vi "ADCP_UI_Continuous_Receiver_Data_Packet_Updater.vi"(8 "error in (no error)":errorcluster, 11 "ADCU_GUI References":T1) -> ()   [LabVIEW 2017]
uses:
  Controls/ADCP_UI/ADCP_UI_Parameters.ctl
  Controls/ADCP_UI/ADCP_UI_Queues.ctl
  Controls/ADCP_UI/ADCP_UI_Continuous_Receiver_States.ctl
  Controls/ADCP_UI/ADCP_Queue_Receive_Log_Queue_Element.ctl
  Controls/Packet/Packet.ctl
  Controls/Packet/Packet_Direction.ctl
  Controls/Packet/Packet_Type.ctl
  Controls/Packet/Packet_Priority.ctl
  Controls/Data Packets/Data_Packet.ctl
  Controls/Data Packets/Parameter.ctl
  Controls/Data Packets/Parameter_Data_Type.ctl
  Controls/Data Packets/Data_Packet_Transmit_Mode.ctl
  Controls/Data Packets/Data_Packet_FGV_Commands.ctl
  ADCP_UI_Receive_List_Data_Packets.vi
panel:
  out "Packet.Frame ID":u8
  out "Packet.Node ID":u8
  out "Process Data":bool
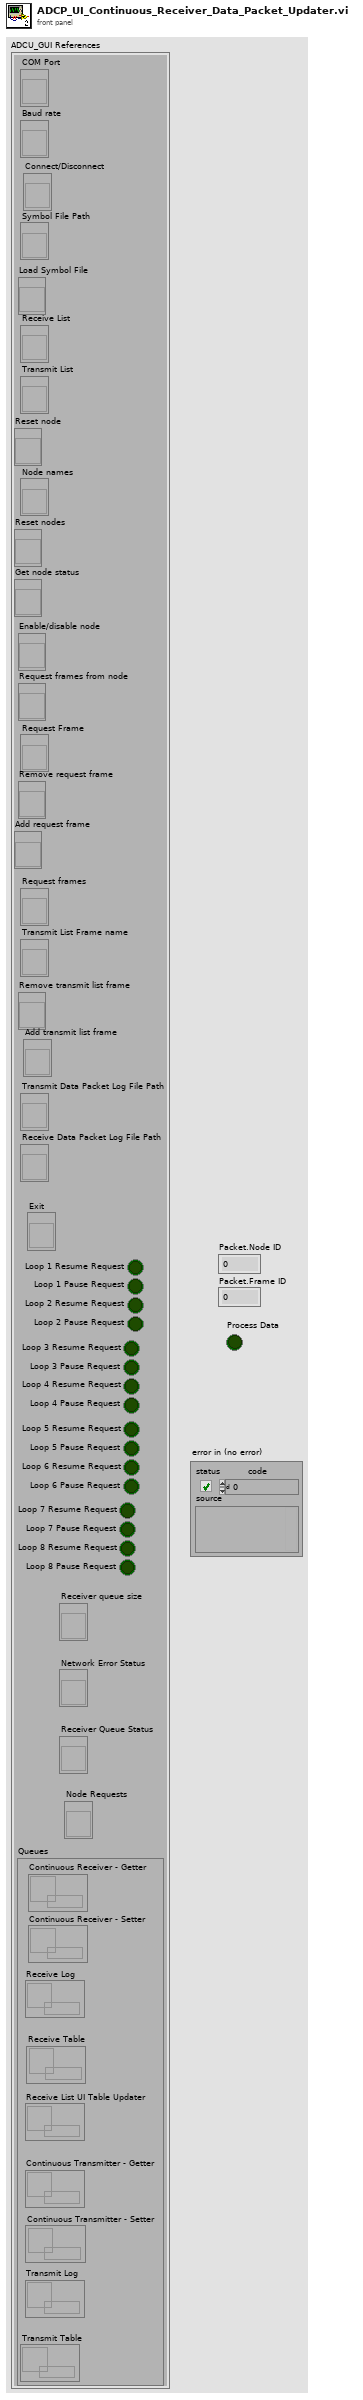
[diagram p1: front panel]
types:
  T1 = typedef "ADCP_UI_Parameters.ctl" = cluster{"COM Port":refnum<vi>, "Baud rate":refnum<vi>, "Symbol File Path":refnum<vi>, "Receive List":refnum<vi>, "Transmit List":refnum<vi>, "Node names":refnum<vi>, "Request Frame":refnum<vi>, "Request frames":refnum<vi>, "Transmit List Frame name":refnum<vi>, "Transmit Data Packet Log File Path":refnum<vi>, "Receive Data Packet Log File Path":refnum<vi>, "Loop 1 Resume Request":bool, "Loop 1 Pause Request":bool, "Loop 2 Resume Request":bool, "Loop 2 Pause Request":bool, "Loop 3 Resume Request":bool, "Loop 3 Pause Request":bool, "Loop 4 Resume Request":bool, "Loop 4 Pause Request":bool, "Loop 5 Resume Request":bool, "Loop 5 Pause Request":bool, "Loop 6 Resume Request":bool, "Loop 6 Pause Request":bool, "Loop 7 Resume Request":bool, "Loop 7 Pause Request":bool, "Loop 8 Resume Request":bool, "Loop 8 Pause Request":bool, "Exit":refnum<vi>, "Connect/Disconnect":refnum<vi>, "Load Symbol File":refnum<vi>, "Reset node":refnum<vi>, "Reset nodes":refnum<vi>, "Get node status":refnum<vi>, "Enable/disable node":refnum<vi>, "Request frames from node":refnum<vi>, "Remove request frame":refnum<vi>, "Add request frame":refnum<vi>, "Remove transmit list frame":refnum<vi>, "Add transmit list frame":refnum<vi>, "Receiver queue size":refnum<vi>, "Network Error Status":refnum<vi>, "Receiver Queue Status":refnum<vi>, "Node Requests":refnum<vi>, "Queues":T2}
  T2 = typedef "ADCP_UI_Queues.ctl" = cluster{"Continuous Receiver - Getter":refnum<queue>, "Continuous Receiver - Setter":refnum<queue>, "Receive Log":refnum<queue>, "Receive Table":refnum<queue>, "Receive List UI Table Updater":refnum<queue>, "Continuous Transmitter - Getter":refnum<queue>, "Continuous Transmitter - Setter":refnum<queue>, "Transmit Log":refnum<queue>, "Transmit Table":refnum<queue>}
  T3 = typedef "Data_Packet_FGV_Commands.ctl" = enum16{"Update all parameters from data packets", "Update Packet", "Load", "Read Packet Parameters", "Write Packet Parameters", "Read Packet Parameter", "Write Packet Parameter", "Read Data Packets", "Read Data Packet", "Read Data Packet by Parameter Name", "Get Parameter Node and Frame ID", "Read Data Packet from Node ID and Frame ID"}
  T4 = typedef "ADCP_Queue_Receive_Log_Queue_Element.ctl" = cluster{"Packet":T5, "Receive Time (ms)":u64, "Count":i32, "Receive Time Interval (ms) ":u64}
  T5 = typedef "Packet.ctl" = cluster{"Raw Bytes":u8[], "Checksum":bool, "Direction":T6, "Processed Bytes":u8[], "Node ID":u8, "Packet type":T7, "Frame Data":u32, "Priority":T8, "Frame ID":u8}
  T6 = typedef "Packet_Direction.ctl" = enum16{"Transmit", "Receive", "Bidirectional"}
  T7 = typedef "Packet_Type.ctl" = enum16{"Data", "Connection Management", "Remote Request", "Error/Status"}
  T8 = typedef "Packet_Priority.ctl" = enum16{"LOW", "HIGH"}
  T9 = typedef "Data_Packet.ctl" = cluster{"Packet":T5, "Parameters":T10[], "Last Received Time (ms)":u64, "Receive count":i32, "Transmit count":i32, "Transmit interval (ms)":u32, "Last Transmitted Time (ms)":u64, "Receive interval (ms)":u32, "Transmit_Mode":T12, "Transmit Enable":bool, "Cyclic Transmit interval (ms)":u32}
  T10 = typedef "Parameter.ctl" = cluster{"Parameter name":string, "Node name":string, "Node ID":u8, "Frame name":string, "Frame ID":u8, "Data type":T11, "Start Bit":i32, "Bit Length":i32, "Factor":dbl, "Offset":dbl, "Minimum":dbl, "Maximum":dbl, "Descriptor":string, "Enum values":string[], "Value":string}
  T11 = typedef "Parameter_Data_Type.ctl" = enum16{"BOOL", "UNSIGNED", "SIGNED", "FLOAT32", "ENUM"}
  T12 = typedef "Data_Packet_Transmit_Mode.ctl" = enum16{"Disabled", "Single", "Cyclic"}
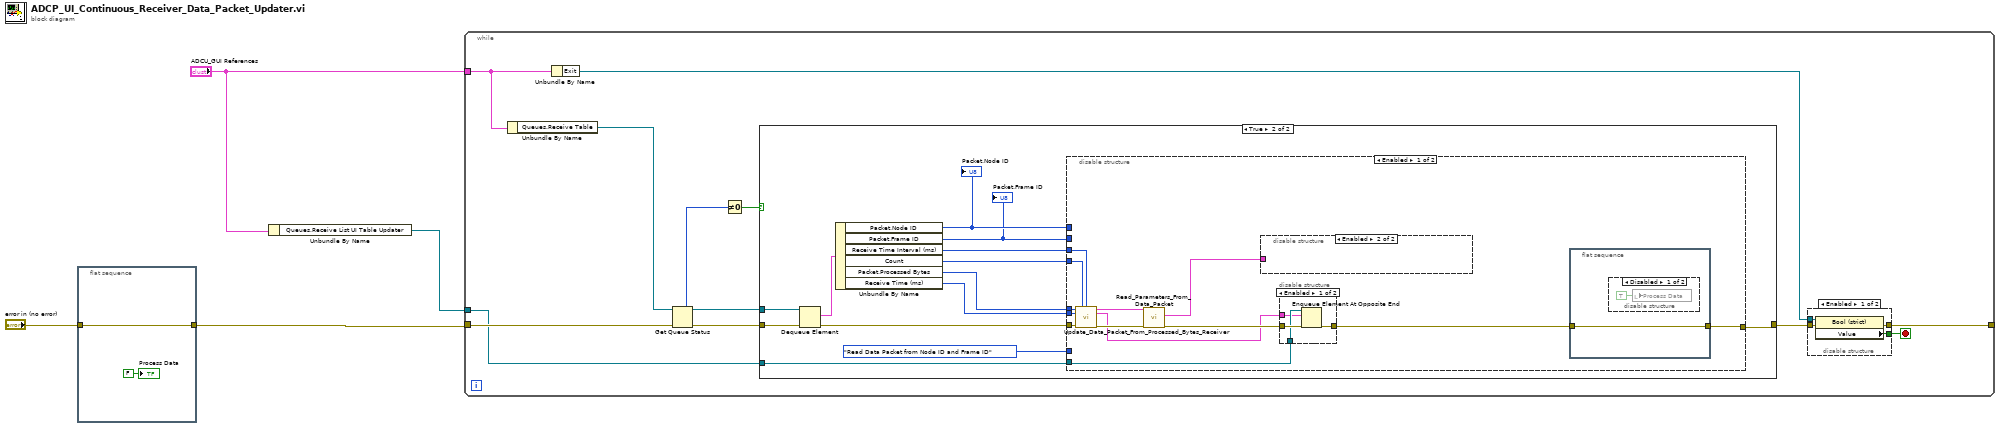
[diagram p0: block diagram]
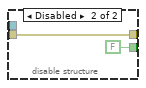
[diagram p2: hidden frame]
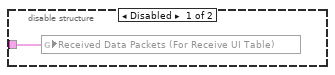
[diagram p4: hidden frame]
diagram:
  n1 = flat-sequence {
    tunnel: "error in (no error)" -> [w6]
    tunnel: [w6] -> w3
    frame #0 {
      "Process Data" <- FALSE ("Process Data")
    }
  }
  n2 = Unbundle By Name("ADCU_GUI References") -> ("Queues.Receive List UI Table Updater"=w1:refnum<queue>)
  n3 = while {
    tunnel: w3 -> [w18]
    tunnel: "ADCU_GUI References" -> [w9]
    tunnel: [w10] -> _
    tunnel: w1 -> [w7]
    stop <- w11 stop-if-true
    n4 = Unbundle By Name(w9) -> ("Queues.Receive Table"=w17:refnum<queue>)
    n5 = Unbundle By Name(w9) -> ("Exit"=w12:refnum<vi>)
    n6 = Get Queue Status(queue=w17, error in (no error)=w18) -> (queue out=w8:refnum<queue>, error out=w15:errorcluster, # elements in queue=w16:i32)  [unwired: 1 in, 5 out]
    n7 = Not Equal To 0?(x=w16) -> (x != 0?=w14:bool)
    n8 = case shown="True" w14 {
      tunnel: w15 -> [w25 w38]
      tunnel: [w25 w27] -> w13
      tunnel: w8 -> [_ w37]
      tunnel: w7 -> [_ w26]
      frame False {
      }
      frame True {
        n9 = Dequeue Element(queue=w37, error in (no error)=w38) -> (element=w35:T4, error out=w36:errorcluster)  [unwired: 1 in, 2 out]
        n10 = Unbundle By Name(w35) -> ("Packet.Node ID"=w29:u8, "Packet.Frame ID"=w28:u8, "Receive Time Interval (ms)"=w31:u64, "Count"=w32:i32, "Packet.Processed Bytes"=w34:u8[], "Receive Time (ms)"=w33:u64)
        "Packet.Node ID" <- w29
        "Packet.Frame ID" <- w28
        n11 = disable-structure shown="Enabled" {
          disable-tunnel: w36 -> [w51 w60]
          disable-tunnel: w34 -> [w50 _]
          disable-tunnel: w33 -> [w49 _]
          disable-tunnel: w32 -> [w48 _]
          disable-tunnel: w31 -> [w47 _]
          disable-tunnel: Data_Packet_FGV_Commands."Read Data Packet from Node ID and Frame ID" ("Commands") -> [_ _]
          disable-tunnel: w29 -> [_ _]
          disable-tunnel: w28 -> [_ _]
          disable-tunnel: [w45 w60] -> w27
          disable-tunnel: w26 -> [w41 _]
          frame Enabled {
            n12 = call "Update_Data_Packet_From_Processed_Bytes_Receiver.vi"("Processed Bytes"=w50, "Receive count"=w48, "Receive interval (ms)"=w47, "Last Receive Time (ms)"=w49, "error in (no error)"=w51) -> ("Updated data packet"=w44:T9, "Data Packets Out"=w40:T9[], "error out"=w46:errorcluster)  [unwired: 8 in]
            n13 = call "Read_Parameters_From_Data_Packet.vi"("error in (no error)"=w46, "Data_Packet in"=w44) -> ("error out"=w43:errorcluster, "Data Packets Out"=w39:T9[])  [unwired: 7 in, 1 out]
            n14 = disable-structure shown="Enabled" {
              disable-tunnel: w39 -> [w52 _]
              frame Disabled {
                n15 = global write "ADCP_UI_Receive_List_Data_Packets.vi" "Received Data Packets (For Receive UI Table)"(w52) -> ()
              }
              frame Enabled {
              }
            }
            n16 = disable-structure shown="Enabled" {
              disable-tunnel: w43 -> [w56 w57]
              disable-tunnel: [w55 w57] -> w42
              disable-tunnel: w41 -> [w54 _]
              disable-tunnel: w40 -> [w53 _]
              frame Enabled {
                n17 = Enqueue Element At Opposite End(queue=w54, element=w53, error in (no error)=w56) -> (error out=w55:errorcluster)  [unwired: 1 in, 2 out]
              }
              frame Disabled {
              }
            }
            n18 = flat-sequence {
              tunnel: w42 -> [w58]
              tunnel: [w58] -> w45
              frame #0 {
                n19 = disable-structure shown="Disabled" {
                  frame Disabled {
                    n20 = local write "Process Data"(TRUE ("Process Data")) -> ()
                  }
                  frame Enabled {
                  }
                }
              }
            }
          }
          frame Disabled {
          }
        }
      }
    }
    n21 = disable-structure shown="Enabled" {
      disable-tunnel: w13 -> [w22 w24]
      disable-tunnel: w12 -> [w21 _]
      disable-tunnel: [w20 FALSE ("Value")] -> w11
      disable-tunnel: [w19 w24] -> w10
      frame Enabled {
        n22 = property class="Bool (strict)"(reference=w21, error in=w22) -> (error out=w19:errorcluster, "Value"=w20:bool)  [unwired: 1 out]
      }
      frame Disabled {
      }
    }
  }
